vi "LAcontroller.vi"() -> ()   [LabVIEW 2016]
uses:
  controls/FPGAVIreferenceTypeDef.ctl
  controls/Enum.ctl
  controls/FPGAVIreferenceTypeDefScanEngine.ctl
  Course Project/support/Message Queue/Message Cluster.ctl
  controls/EnumFGVHDT.ctl
  <vilib>/rvi/errors/niLvFpgaAdjustHostInterfaceError.vi
  <vilib>/rvi/interface/common/niFpgaWaitOnOcc.vi
  <vilib>/regexp/Match Regular Expression.xnode
  <vilib>/rvi/interface/nirviReadWriteControl/nirviReadWriteControl.xnode
  FPGA Bitfiles/qnmController797_usbRIO_controllerFPGAmu.lvbitx
  <vilib>/rvi/interface/nirviMethod/nirviMethod.xnode
  Course Project/support/Message Queue/Message Queue.lvlib
  <vilib>/rvi/errors/niLvFpgaMergeErrorWithErrorCode.vi
  NiFpgaLv.dll
  <vilib>/FPGAPlugInAG/USB-7856R OEM/niLvFpga_ConfigureFifo_USB-7856R OEM.vi
  <vilib>/FPGAPlugInAG/USB-7856R OEM/niLvFpga_ReadFifo_USB-7856R OEM.vi
panel:
  in  "disable Filters":bool
  out "Warning":string
  in  "setUnityFilters":bool
  out "idSourceName":string
  in  "Identification Type":T1
  out "axialFiltersLoaded":bool
  out "lateralFiltersLoaded":bool
  out "Nominal Response Phi":cluster{dbl[], dbl[]}[](graph)
  out "Nominal Response A":cluster{dbl[], dbl[]}[](graph)
  out "Measured Resp Phi":cluster{dbl[], dbl[]}(graph)
  out "Measured Resp A":cluster{dbl[], dbl[]}(graph)
  out "Time domain":i16[][](graph)
  out "acquisitionDone":dbl(slide) scale=0.0..1.0
  out "Message":string="Exit"
  in  "Filtering mode":enum16{"Axial", "Lateral"}(ring)
  in  "Controller Order":dbl=10.0 min=2.0 max=16.0 step=2.0
  in  "Save identification":bool
  in  "resetFilters":bool
  out "Sampling Frequency":dbl=686813.0 format="%#_4p"
  in  "clearBuffer":bool
  in  "System ID Parameters":T2={"Output Decimation"=1, "Repetitions"=100, "PRBS Order"=12, "low Value"=0.0, "high Value"=0.0005035400390625} {"high Value" format="%#_3p"; "Output Decimation" min=1}
  in  "doControlDesign":bool
  in  "Desired bandwidth":dbl=7000.0 min=500.0 format="%#_13pHz"
  out "Ki":dbl format="%#_3p"
  out "Kp":dbl format="%#_3p"
  out "PRBS length":u16=8191
  # "System Settings"
  # "Control Design"
  # "Measured System Response"
  # "Nominal System Response"
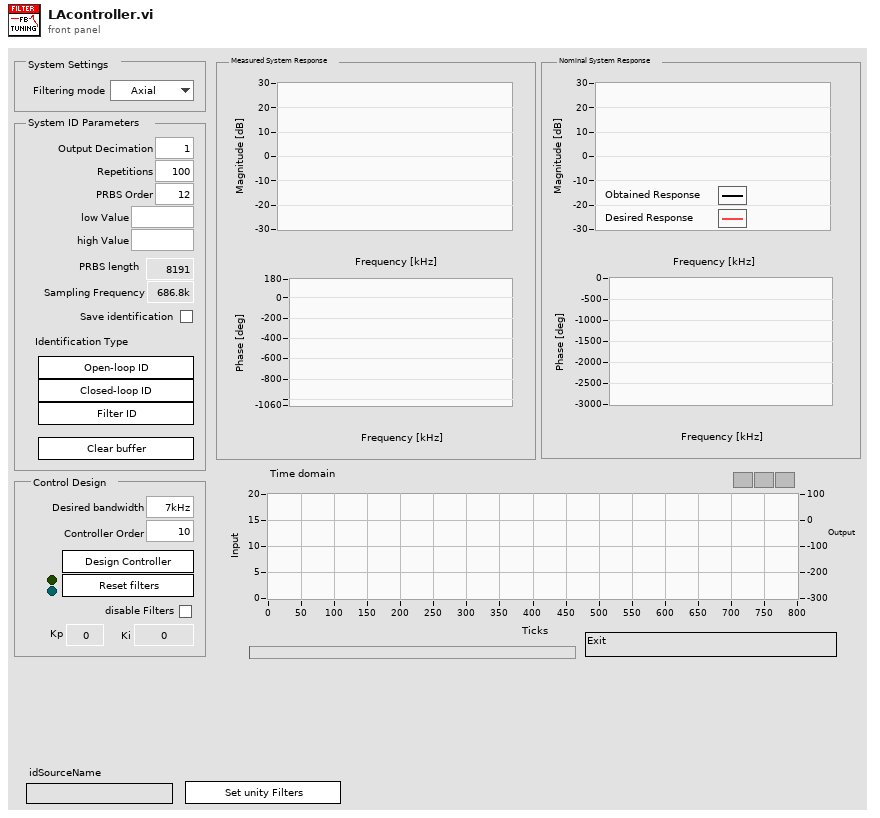
[diagram p1: front panel]
types:
  T1 = cluster{"Error":bool, "Height":bool, "Filter":bool}
  T2 = cluster{"Output Decimation":u16, "Repetitions":u16, "PRBS Order":u16, "low Value":fxp<+/-,17,1>, "high Value":fxp<+/-,17,1>}
  T3 = typedef "Message Queue.lvlib/All Message Queues.ctl" = cluster{"IU":refnum<queue>}
  T4 = cluster{"OldVal":enum16{"Axial", "Lateral"}, "NewVal":enum16{"Axial", "Lateral"}}
  T5 = typedef "eventsource.ctl" = u32
  T6 = cluster{"openLoopID":bool, "closedLoopID":bool, "filterID":bool}
  T7 = typedef "FPGAVIreferenceTypeDefScanEngine.ctl" = refnum<k20>
  T8 = typedef "Enum.ctl" = enum16{"Init", "Read", "Write"}
  T9 = typedef "FPGAVIreferenceTypeDef.ctl" = refnum<k20>
  T10 = cluster{"Output Decimation":u16, "Repetitions":u16, "PRBS Order":u16, "low Value":fxp<+/-,17,1>, "high Value":fxp<+/-,17,1>}[]
  T11 = typedef "Message Queue.lvlib/Message Cluster.ctl" = cluster{"Message":string, "Données de message":variant}
  T12 = cluster{"sysIdOutputRate":u16, "sysIdWaveSize":u16, "sysIdRepetitions":u16, "lowValue":fxp<+/-,16,1>, "highValue":fxp<+/-,16,1>}
  T13 = typedef "EnumFGVHDT.ctl" = enum16{"Init", "Read", "Write", "Push", "Pop"}
  T14 = cluster{"OwnerVi":string, "hdt.int.s.transferSource":u8, "Used":bool}
  T15 = cluster{"scanEngineHz":u32, "feedbackHz":u32, "sicmHz":u32, "rampHz":u32}
  T16 = cluster{"hdt.int.s.transferSource":u8, "hdt.int.p.useInternalMemStartPos":bool, "hdt.int.p.memStartPos":fxp<+,14,14>, "hdt.int.p.readLength":u16, "hdt.int.p.readFwd":bool, "hdt.int.p.memReadDec":u16, "hdt.int.p.startTransfer":bool}
  T17 = cluster{"System ID Parameters":cluster{"Output Decimation":u16, "Repetitions":u16, "PRBS Order":u16, "low Value":fxp<+/-,17,1>, "high Value":fxp<+/-,17,1>}, "PRBS length":u16, "Sampling Frequency":dbl, "flt.p.b8x":fxp<+/-,24,8>[], "flt.p.anot8x":fxp<+/-,24,8>[], "flt.bypass1":bool[]}
  T18 = typedef "imagedata.ctl" = cluster{"image type":i32, "image depth":i32, "image":u8[], "mask":u8[], "colors":u32[], "Rectangle":cluster{"left":i16, "top":i16, "right":i16, "bottom":i16}}
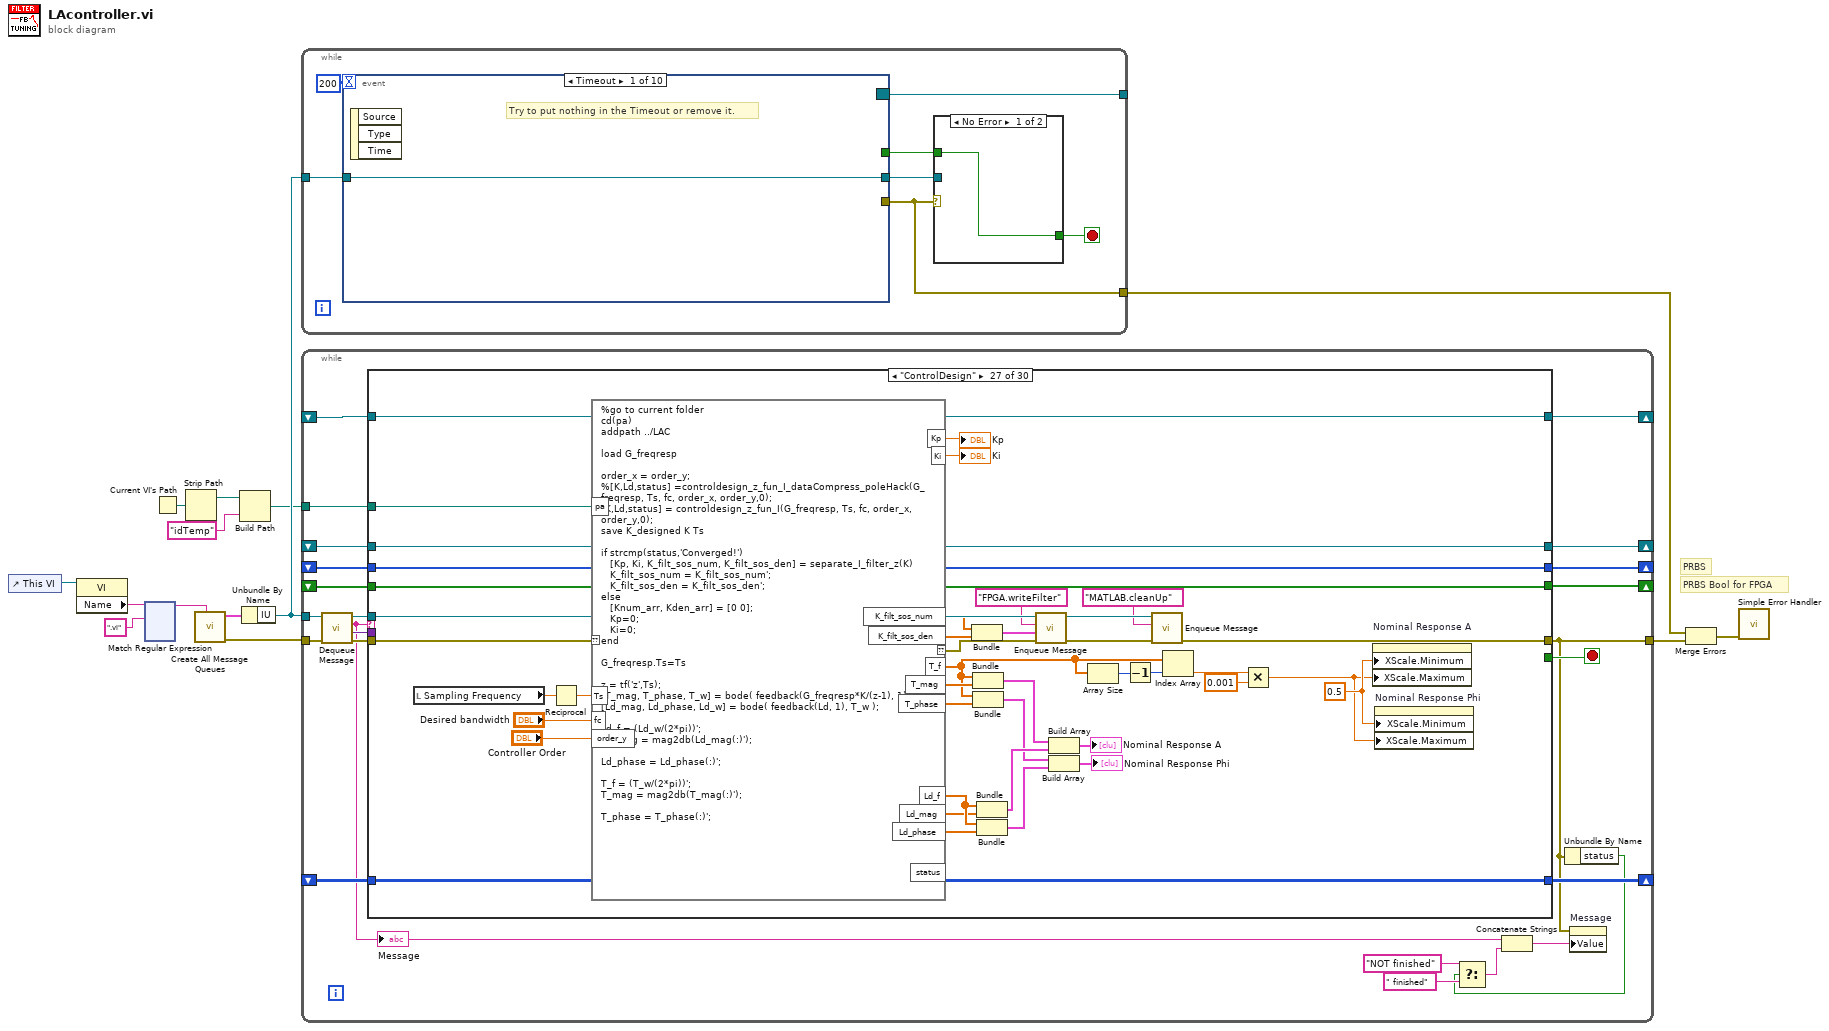
[diagram p0: block diagram]
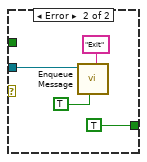
[diagram p2: hidden frame]
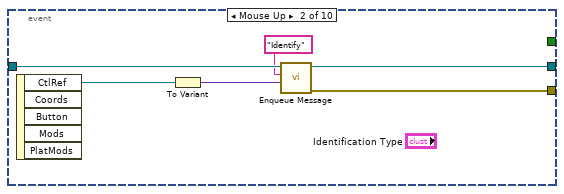
[diagram p3: hidden frame]
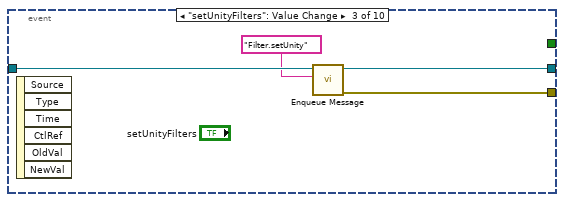
[diagram p4: hidden frame]
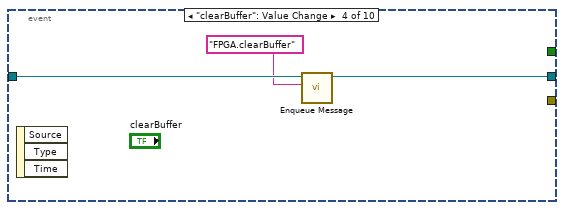
[diagram p5: hidden frame]
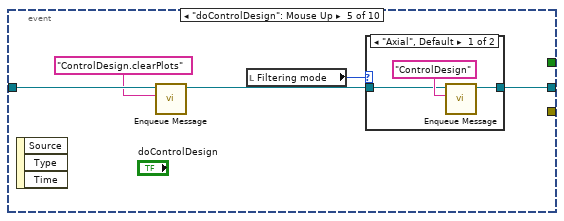
[diagram p6: hidden frame]
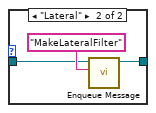
[diagram p7: hidden frame]
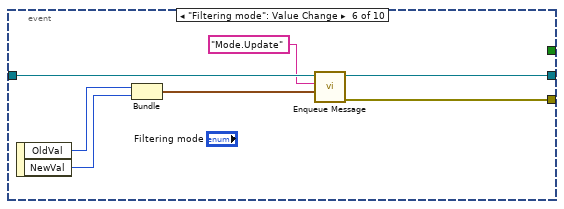
[diagram p8: hidden frame]
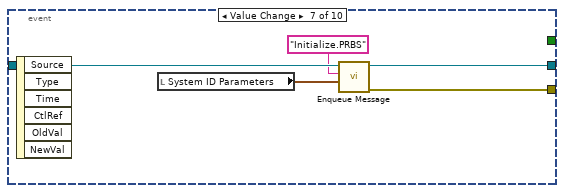
[diagram p9: hidden frame]
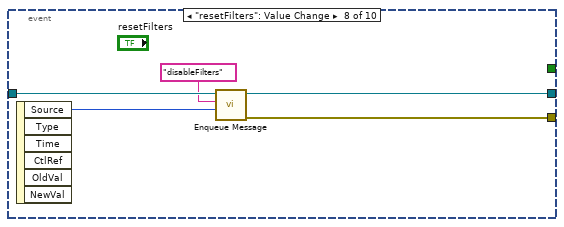
[diagram p10: hidden frame]
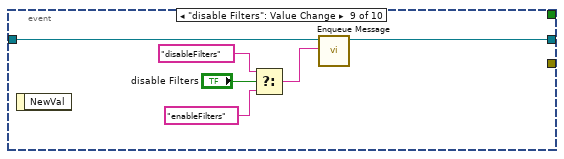
[diagram p11: hidden frame]
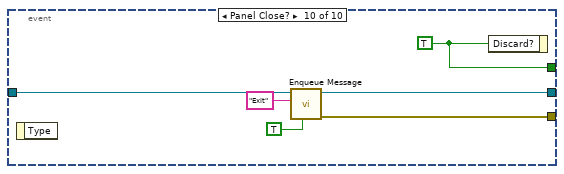
[diagram p12: hidden frame]
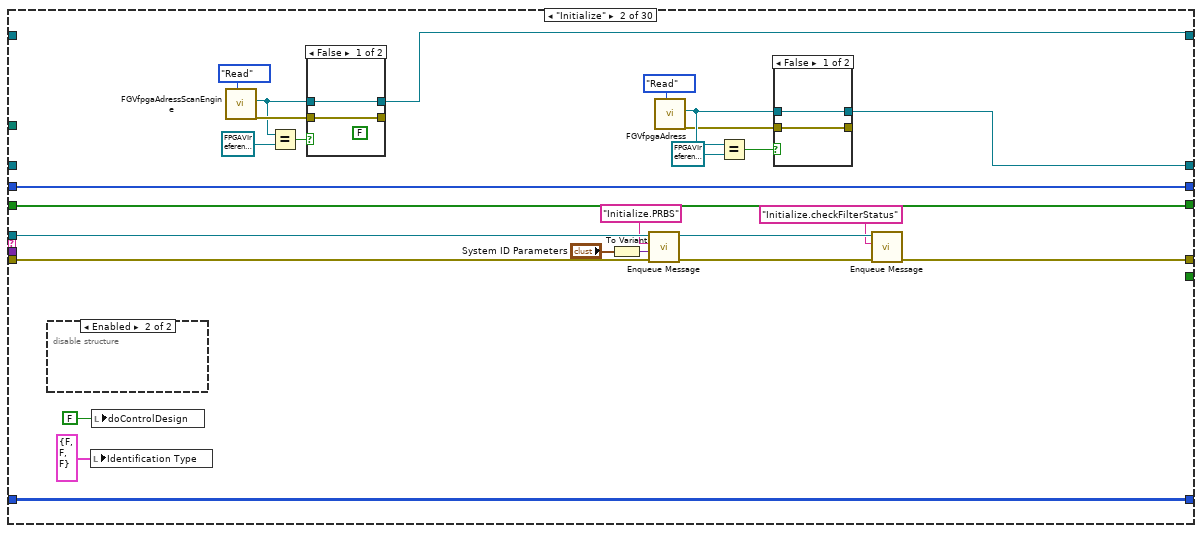
[diagram p14: hidden frame]
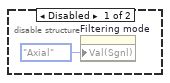
[diagram p15: hidden frame]
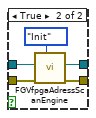
[diagram p16: hidden frame]
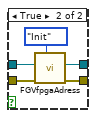
[diagram p17: hidden frame]
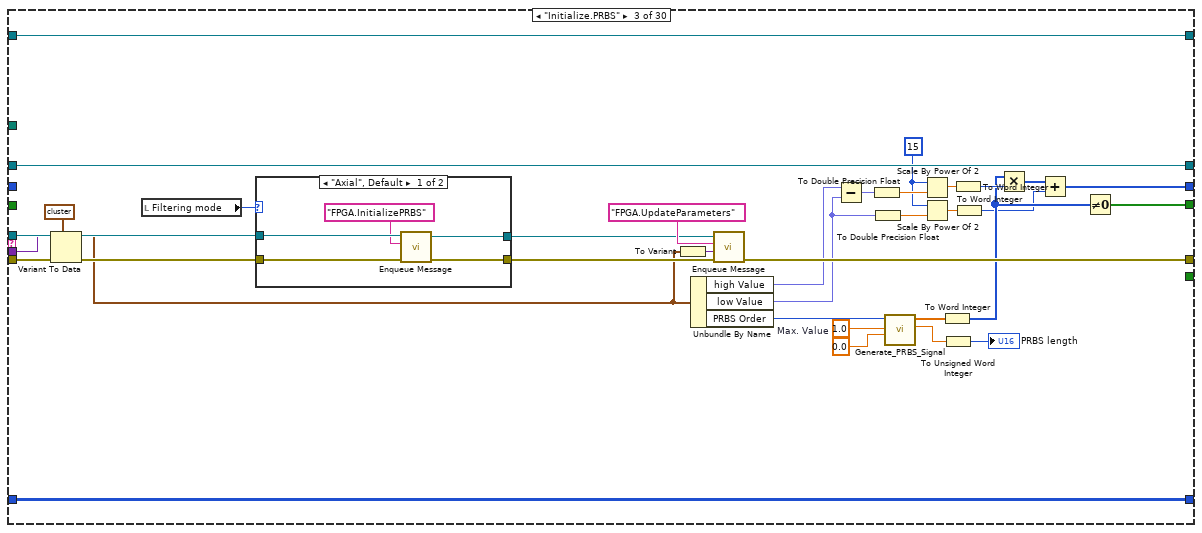
[diagram p18: hidden frame]
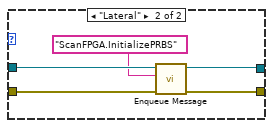
[diagram p19: hidden frame]
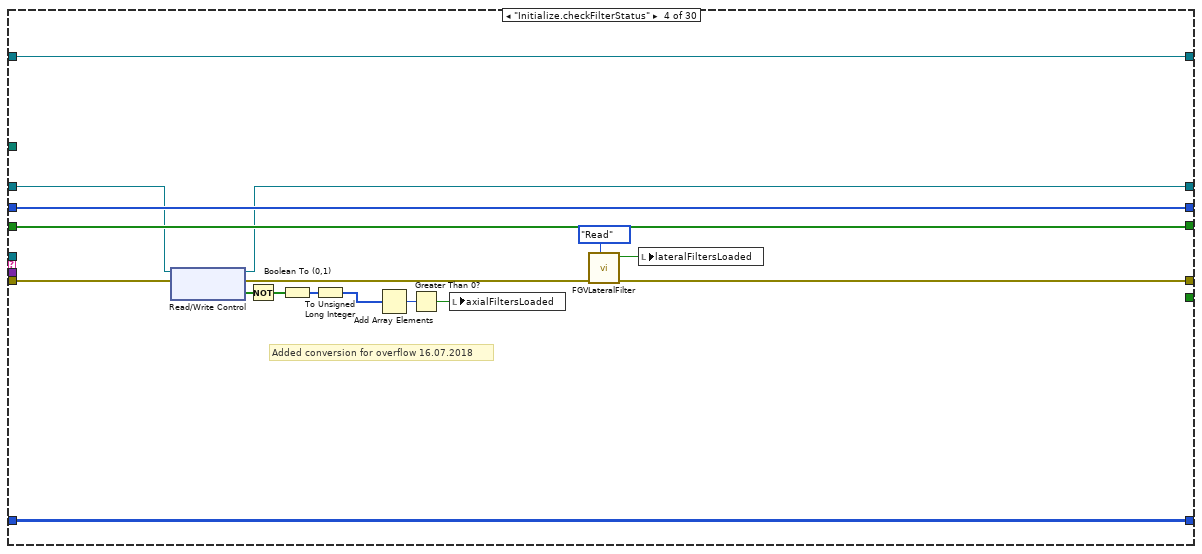
[diagram p20: hidden frame]
diagram:
  # "PRBS Bool for FPGA"
  # "PRBS"
  n1 = control-ref of="This VI"() -> (w4:refnum<vi>)
  n2 = property class="VI"(reference=w4) -> ("Name"=w3:string)  [unwired: 1 in, 2 out]
  n3 = xnode "Match Regular Expression"("input string"=w3, "regular expression"=".vi") -> ("before match"=w1:string)  [unwired: 4 in, 4 out]
  n4 = Current VI's Path() -> (path=w8:path)
  n5 = Strip Path(path=w8) -> (stripped path=w6:path)  [unwired: 1 out]
  n6 = call "Create All Message Queues.vi"("QueueName"=w1) -> ("ErrorOut"=w12:errorcluster, "MessageQueueOut"=w14:T3)  [unwired: 9 in]
  n7 = Build Path(base path=w6, name or relative path="idTemp") -> (appended path=w5:path)
  n8 = Unbundle By Name(w14) -> ("IU"=w13:refnum<queue>)
  n9 = while {
    tunnel: w13 -> [w21]
    tunnel: [w17] -> w9
    tunnel: [w16] -> _
    stop <- w19 stop-if-true
    n10 = event shown="[0] Timeout" {
      selector: _ -> [_ _ _ _ _ _ _ _ _ _]
      dyn-events: [_ _ _ _ _ _ _ _ _ _] -> w16
      timeout: 200 -> [_ _ _ _ _ _ _ _ _ _]
      tunnel: [_ _ _ _ _ _ _ _ _ w80] -> w20
      tunnel: w21 -> [w27 w33 w37 w40 w43 w58 w63 w68 w74 w79]
      tunnel: [_ w28 w35 _ _ w52 w62 w66 _ w78] -> w17
      tunnel: [w27 w29 w36 w39 w45 w53 w60 w64 w73 w77] -> w18
      event Timeout {
        # "Try to put nothing in the Timeout or remove it."
        n11 = event-data() -> ()  [unwired: 1 in, 3 out]
      }
      event "Identification Type.Error", "Identification Type.Height", "Identification Type.Filter": Mouse Up {
        n12 = event-data() -> ("CtlRef"=w31:refnum<vi>)  [unwired: 1 in, 4 out]
        n13 = To Variant(anything=w31) -> (Variant=w30:variant)
        n14 = call "Enqueue Message.vi"("Data"=w30, "Message"="Identify", "Queue"=w33) -> ("error out"=w28:errorcluster, "Queue dup."=w29:refnum<queue>)  [unwired: 7 in]
      }
      event "setUnityFilters": Value Change {
        n15 = event-data() -> ()  [unwired: 1 in, 6 out]
        n16 = call "Enqueue Message.vi"("Message"="Filter.setUnity", "Queue"=w37) -> ("error out"=w35:errorcluster, "Queue dup."=w36:refnum<queue>)  [unwired: 8 in]
      }
      event "clearBuffer": Value Change {
        n17 = event-data() -> ()  [unwired: 1 in, 3 out]
        n18 = call "Enqueue Message.vi"("Message"="FPGA.clearBuffer", "Queue"=w40) -> ("Queue dup."=w39:refnum<queue>)  [unwired: 8 in, 1 out]
      }
      event "doControlDesign": Mouse Up {
        n19 = event-data() -> ()  [unwired: 1 in, 3 out]
        n20 = call "Enqueue Message.vi"("Message"="ControlDesign.clearPlots", "Queue"=w43) -> ("Queue dup."=w42:refnum<queue>)  [unwired: 8 in, 1 out]
        n21 = local read "Filtering mode"() -> (w44:enum16{"Axial", "Lateral"})
        n22 = case shown="\"Axial\", Default" w44 {
          tunnel: w42 -> [w47 w50]
          tunnel: [w46 w49] -> w45
          frame "Axial", Default {
            n23 = call "Enqueue Message.vi"("Message"="ControlDesign", "Queue"=w47) -> ("Queue dup."=w46:refnum<queue>)  [unwired: 8 in, 1 out]
          }
          frame "Lateral" {
            n24 = call "Enqueue Message.vi"("Message"="MakeLateralFilter", "Queue"=w50) -> ("Queue dup."=w49:refnum<queue>)  [unwired: 8 in, 1 out]
          }
        }
      }
      event "Filtering mode": Value Change {
        n25 = event-data() -> ("OldVal"=w55:enum16{"Axial", "Lateral"}, "NewVal"=w56:enum16{"Axial", "Lateral"})  [unwired: 1 in]
        n26 = Bundle("OldVal"=w55, "NewVal"=w56) -> (w54:T4)  [unwired: 1 in]
        n27 = call "Enqueue Message.vi"("Data"=w54, "Message"="Mode.Update", "Queue"=w58) -> ("error out"=w52:errorcluster, "Queue dup."=w53:refnum<queue>)  [unwired: 7 in]
      }
      event "System ID Parameters.PRBS Order": Value Change {
        n28 = event-data() -> ()  [unwired: 1 in, 6 out]
        n29 = local read "System ID Parameters"() -> (w59:T2)
        n30 = call "Enqueue Message.vi"("Data"=w59, "Message"="Initialize.PRBS", "Queue"=w63) -> ("error out"=w62:errorcluster, "Queue dup."=w60:refnum<queue>)  [unwired: 7 in]
      }
      event "resetFilters": Value Change {
        n31 = event-data() -> ("Source"=w67:T5)  [unwired: 1 in, 5 out]
        n32 = call "Enqueue Message.vi"("Data"=w67, "Message"="disableFilters", "Queue"=w68) -> ("error out"=w66:errorcluster, "Queue dup."=w64:refnum<queue>)  [unwired: 7 in]
      }
      event "disable Filters": Value Change {
        n33 = event-data() -> ()  [unwired: 1 in, 1 out]
        n34 = Select(t="disableFilters", s="disable Filters", f="enableFilters") -> (s? t:f=w72:string)
        n35 = call "Enqueue Message.vi"("Message"=w72, "Queue"=w74) -> ("Queue dup."=w73:refnum<queue>)  [unwired: 8 in, 1 out]
      }
      event Panel Close? {
        w80 = TRUE ("Rejeter ?")
        n36 = event-data() -> ()  [unwired: 1 in, 1 out]
        n37 = call "Enqueue Message.vi"("Prioritary message"=TRUE ("Message prioritaire ? (F)"), "Message"="Exit", "Queue"=w79) -> ("error out"=w78:errorcluster, "Queue dup."=w77:refnum<queue>)  [unwired: 7 in]
        n38 = event-data ("Event Filter Node")("Discard?"=w80) -> ()  [unwired: 1 in, 1 out]
      }
    }
    n39 = case shown="No Error" w17 {
      tunnel: [w22 TRUE ("Rejeter ?")] -> w19
      tunnel: w20 -> [w22 _]
      tunnel: w18 -> [_ w25]
      frame No Error {
      }
      frame Error {
        n40 = call "Enqueue Message.vi"("Prioritary message"=TRUE ("Message prioritaire ? (F)"), "Message"="Exit", "Queue"=w25) -> ()  [unwired: 7 in, 2 out]
      }
    }
  }
  n41 = while {
    tunnel: w13 -> [w99]
    tunnel: w12 -> [w103]
    tunnel: [w85] -> w10
    shift-right: [w97] -> _
    shift-left: _ -> [w98]
    shift-right: [w96] -> _
    shift-left: _ -> [w95]
    shift-right: [w94] -> _
    shift-left: _ -> [w93]
    shift-right: [w91] -> _
    shift-left: _ -> [w92]
    shift-right: [w90] -> _
    shift-left: _ -> [w89]
    tunnel: w5 -> [w88]
    stop <- w104 stop-if-true
    n42 = call "Dequeue Message.vi"("entrée d'erreur (pas d'erreur)"=w103, "File d'attente de messages"=w99) -> ("sortie d'erreur"=w102:errorcluster, "Données de message"=w101:variant, "Message"=w87:string, "File d'attente de message dup."=w100:refnum<queue>)  [unwired: 6 in]
    "Message" <- w87
    n43 = case "Conditions des messages" shown="\"ControlDesign\"" w87 {
      selector: w87 -> [_ _ _ _ _ _ _ _ _ _ _ _ _ _ _ _ _ _ _ _ _ _ _ _ _ _ _ _ _ w1015]
      tunnel: w100 -> [_ w133 w184 _ _ w235 w254 w341 w365 _ _ _ _ _ _ _ _ _ _ _ _ _ w793 _ _ _ w970 _ w1006 _]
      tunnel: w102 -> [w110 w132 w181 w209 w219 w234 w261 w336 w353 w373 w385 w404 w428 w451 w520 w550 w592 w630 w689 w718 w728 w752 w760 w831 w879 w927 w935 w995 w1004 _]
      tunnel: [w110 w114 w185 w200 w219 w223 w280 w323 w352 w373 w375 w400 w438 w459 w527 w547 w591 w631 w654 w702 w731 w752 w761 w830 w868 w927 w931 w995 w1003 w1013] -> w85
      tunnel: [_ _ _ _ _ _ _ _ _ _ _ _ _ _ _ _ _ _ _ _ _ _ _ _ _ _ _ _ TRUE _] -> w104
      tunnel: w101 -> [_ _ w180 _ _ w229 _ w335 _ _ _ w403 _ _ w519 w549 _ _ w690 _ _ _ w775 _ w878 _ _ _ _ _]
      tunnel: w98 -> [w109 _ w171 w208 w218 w233 w283 w322 w364 w372 w381 w402 w437 w465 w516 w545 w594 w628 w679 w717 w733 w751 w812 w836 w852 w926 w969 w994 w1002 w1011]
      tunnel: [w109 w117 w171 w207 w218 w233 w283 w321 w364 w372 w374 w401 w436 w460 w526 w544 w593 w629 w675 w704 w732 w751 w812 w836 w852 w926 w969 w994 w1002 w1011] -> w97
      tunnel: [w108 w136 w168 w213 w217 w232 w287 w340 w363 w371 w377 w415 w430 w464 w525 w553 w590 w627 w693 w722 w735 w750 w811 w835 w885 w925 w968 w993 w1001 w1010] -> w96
      tunnel: w95 -> [w108 w136 _ w213 w217 w232 w287 w340 w363 w371 w377 w415 w430 w464 w525 w553 w590 w627 w693 w722 w735 w750 w811 w835 w885 w925 w968 w993 w1001 w1010]
      tunnel: [w107 w135 w182 w212 w216 w222 w279 w339 w362 w370 w384 w414 w433 w463 w524 w552 w588 w625 w692 w721 w734 w749 w810 w834 w884 w924 w967 w992 w1000 w1009] -> w94
      tunnel: w93 -> [w107 w135 w182 w212 w216 w222 w279 w339 w362 w370 w384 w414 w433 w463 w524 w552 _ _ w692 w721 w734 w749 w810 w834 w884 w924 w967 w992 w1000 w1009]
      tunnel: w92 -> [w106 _ w177 w211 w215 w231 w278 w338 w361 w369 w380 w398 w440 w462 w522 w543 w587 w637 w681 w720 w730 w748 w813 w833 w883 w923 w942 w990 w998 w1008]
      tunnel: [w106 w118 w177 w211 w215 w231 w278 w338 w361 w369 w380 w397 w439 w462 w521 w543 w587 w637 w681 w720 w730 w748 w813 w833 w883 w923 w942 w990 w998 w1008] -> w91
      tunnel: [w105 w134 w170 w210 w214 w230 w286 w337 w360 w368 w378 w413 w431 w461 w523 w551 w595 w636 w680 w719 w729 w747 w797 w832 w882 w922 w941 w989 w999 w1007] -> w90
      tunnel: w89 -> [w105 w134 _ w210 w214 w230 w286 w337 w360 w368 w378 w413 w431 w461 w523 w551 w595 w636 w680 w719 w729 w747 w797 w832 w882 w922 w941 w989 w999 w1007]
      tunnel: w88 -> [_ _ _ _ _ _ _ _ _ _ _ _ _ _ _ _ _ _ _ _ _ _ w791 _ w860 _ w937 w972 _ _]
      frame "--------- Initialization ---------" {
      }
      frame "Initialize" {
        n44 = disable-structure shown="Enabled" {
          frame Disabled {
            n45 = property on="Filtering mode" class="Enum (strict)"("Val(Sgnl)"=enum16{"Axial", "Lateral"}."Axial" ("Filtering mode")) -> ()  [unwired: 2 in, 2 out]
          }
          frame Enabled {
          }
        }
        n46 = local write "Identification Type"(T6 {"openLoopID"=FALSE, "closedLoopID"=FALSE, "filterID"=FALSE} ("Identification Type")) -> ()
        n47 = local write "doControlDesign"(FALSE ("doLatFilterDesign")) -> ()
        n48 = call "FGVfpgaAdressScanEngine.vi"("Enum"=Enum."Read") -> ("error out"=w127:errorcluster, "FPGA.SEout"=w125:T7)  [unwired: 6 in, 3 out]
        n49 = Equal?(x=w125, y=T7 refnum ("FPGA.SEout")) -> (x = y?=w126:bool)
        n50 = case shown="False" w126 {
          tunnel: [w139 w144] -> w118
          tunnel: [w138 w143] -> _
          tunnel: w127 -> [w138 w142]
          tunnel: w125 -> [w139 w141]
          frame False {
            (unwired) FALSE
          }
          frame True {
            n51 = call "FGVfpgaAdressScanEngine.vi"("Enum"=Enum."Init", "error in"=w142, "FPGA.SEin"=w141) -> ("error out"=w143:errorcluster, "FPGA.SEout"=w144:T7)  [unwired: 4 in, 3 out]
          }
        }
        n52 = To Variant(anything="System ID Parameters") -> (Variant=w111:variant)
        n53 = call "Enqueue Message.vi"("error in"=w132, "Data"=w111, "Message"="Initialize.PRBS", "Queue"=w133) -> ("error out"=w115:errorcluster, "Queue dup."=w116:refnum<queue>)  [unwired: 6 in]
        n54 = call "FGVfpgaAdress.vi"("Enum"=Enum."Read") -> ("error out"=w119:errorcluster, "FPGA VI Reference Out"=w121:T9)  [unwired: 5 in, 4 out]
        n55 = Equal?(x=w121, y=T9 refnum ("FPGA VI Reference Out")) -> (x = y?=w120:bool)
        n56 = case shown="False" w120 {
          tunnel: [w146 w151] -> w117
          tunnel: [w145 w150] -> _
          tunnel: w119 -> [w145 w149]
          tunnel: w121 -> [w146 w148]
          frame False {
          }
          frame True {
            n57 = call "FGVfpgaAdress.vi"("Enum"=Enum."Init", "error in"=w149, "FPGA VI Reference In"=w148) -> ("error out"=w150:errorcluster, "FPGA VI Reference Out"=w151:T9)  [unwired: 3 in, 4 out]
          }
        }
        n58 = call "Enqueue Message.vi"("error in"=w115, "Message"="Initialize.checkFilterStatus", "Queue"=w116) -> ("error out"=w114:errorcluster)  [unwired: 7 in, 1 out]
      }
      frame "Initialize.PRBS" {
        w159 = i16 15 ("n")
        w178 = 1.0  # Max. Value
        n59 = Variant To Data(error in=w181, type=T2 {"Output Decimation"=1, "Repetitions"=1000, "PRBS Order"=12, "low Value"=0.0, "high Value"=0.0005035400390625} ("System ID Parameters"), Variant=w180) -> (data=w154:T2, error out=w164:errorcluster)
        n60 = local read "Filtering mode"() -> (w153:enum16{"Axial", "Lateral"})
        n61 = case shown="\"Axial\", Default" w153 {
          tunnel: [w191 w193] -> w186
          tunnel: w184 -> [w190 w196]
          tunnel: [w189 w194] -> w152
          tunnel: w164 -> [w187 w192]
          frame "Axial", Default {
            n62 = call "Enqueue Message.vi"("error in"=w187, "Message"="FPGA.InitializePRBS", "Queue"=w190) -> ("error out"=w191:errorcluster, "Queue dup."=w189:refnum<queue>)  [unwired: 7 in]
          }
          frame "Lateral" {
            n63 = call "Enqueue Message.vi"("error in"=w192, "Message"="ScanFPGA.InitializePRBS", "Queue"=w196) -> ("error out"=w193:errorcluster, "Queue dup."=w194:refnum<queue>)  [unwired: 7 in]
          }
        }
        n64 = To Variant(anything=w154) -> (Variant=w155:variant)
        n65 = Unbundle By Name(w154) -> ("high Value"=w173:fxp<+/-,17,1>, "low Value"=w161:fxp<+/-,17,1>, "PRBS Order"=w160:u16)
        n66 = call "Enqueue Message.vi"("error in"=w186, "Data"=w155, "Message"="FPGA.UpdateParameters", "Queue"=w152) -> ("error out"=w185:errorcluster)  [unwired: 6 in, 1 out]
        n67 = Subtract(x=w173, y=w161) -> (x-y=w176:fxp<+/-,18,2>)
        n68 = To Double Precision Float(number=w176) -> (double precision float=w162:dbl)
        n69 = To Double Precision Float(number=w161) -> (double precision float=w163:dbl)
        n70 = call "Generate_PRBS_Signal.vi"("Min.Value"=0.0, "Max. Value"=w178, "PRBS Order"=w160) -> ("PRBS Signal Length"=w169:dbl, "PRBS Signal"=w183:dbl[])  [unwired: 7 in]
        n71 = Scale By Power Of 2(n=w159, x=w162) -> (x*2^n=w175:dbl)
        n72 = Scale By Power Of 2(n=w159, x=w163) -> (x*2^n=w167:dbl)
        n73 = To Word Integer(number=w183) -> (16bit integer=w172:i16[])
        n74 = To Unsigned Word Integer(number=w169) -> (unsigned 16bit integer=→"PRBS length":u16)
        n75 = To Word Integer(number=w175) -> (16bit integer=w174:i16)
        n76 = To Word Integer(number=w167) -> (16bit integer=w166:i16)
        n77 = Multiply(x=w172, y=w174) -> (x*y=w165:i16[])
        n78 = Add(x=w165, y=w166) -> (x+y=w168:i16[])
        n79 = Not Equal To 0?(x=w172) -> (x != 0?=w170:bool[])
      }
      frame "Initialize.checkFilterStatus" {
        # "Added conversion for overflow 16.07.2018"
        n80 = xnode "Read/Write Control"("FPGA VI Reference In"=w208, "error in"=w209) -> ("FPGA VI Reference Out"=w207:T9, "error out"=w201:errorcluster, "flt.bypass1"=w206:bool[])
        n81 = Not(x=w206) -> (.not. x?=w204:bool[])
        n82 = Boolean To (0,1)(Boolean=w204) -> (0, 1=w205:i16[])
        n83 = To Unsigned Long Integer(number=w205) -> (unsigned 32bit integer=w197:u32[])
        n84 = Add Array Elements(numeric array=w197) -> (sum=w203:u32)
        n85 = Greater Than 0?(x=w203) -> (x > 0?=w202:bool)
        n86 = local write "axialFiltersLoaded"(w202) -> ()
        n87 = call "FGVLateralFilter.vi"("Enum"=Enum."Read", "error in"=w201) -> ("error out"=w200:errorcluster, "Filter valid output"=w198:bool)  [unwired: 5 in, 1 out]
        n88 = local write "lateralFiltersLoaded"(w198) -> ()
      }
      frame "--- Modal ----" {
      }
      frame "Mode.Update" {
        n89 = Variant To Data(type=T4 {"OldVal"=enum."Axial", "NewVal"=enum."Axial"} ("output cluster"), Variant=w229) -> (data=w227:T4)  [unwired: 1 in, 1 out]
        n90 = local read "System ID Parameters"() -> (w221:T2)
        n91 = local read "Desired bandwidth"() -> (w220:dbl)
        n92 = Unbundle(w227) -> ("OldVal"=w225:enum16{"Axial", "Lateral"}, "NewVal"=w224:enum16{"Axial", "Lateral"})
        n93 = Not Equal?(x=w225, y=w224) -> (x != y?=w226:bool)
        n94 = case shown="True" w226 {
          tunnel: w225 -> [_ w239]
          tunnel: w224 -> [_ w252]
          tunnel: w234 -> [w236 w249]
          tunnel: [w236 w248] -> w223
          tunnel: w235 -> [_ w251]
          tunnel: w221 -> [_ w238]
          tunnel: w220 -> [_ w237]
          frame False {
          }
          frame True {
            # "Initial desired frequencies"
            # "Initial sysID params"
            n95 = feedback #1(T10 [{"Output Decimation"=1, "Repetitions"=100, "PRBS Order"=12, "low Value"=0.0, "high Value"=0.00140380859375}, {"Output Decimation"=80, "Repetitions"=100, "PRBS Order"=12, "low Value"=0.0, "high Value"=0.0005035400390625}]) -> (w244:T10)
            n96 = Replace Array Subset(array=w244, new element=w238, index=w239) -> (w245:T10)
            n97 = feedback-in #1(w245) -> ()
            n98 = Index Array(array=w244, index=w252) -> (element=w247:T2)
            n99 = local write "System ID Parameters"(w247) -> ()
            n100 = call "Enqueue Message.vi"("error in"=w249, "Data"=w247, "Message"="Initialize.PRBS", "Queue"=w251) -> ("error out"=w248:errorcluster)  [unwired: 6 in, 1 out]
            n101 = feedback #2(dbl[] [8000.0, 1000.0]) -> (w243:dbl[])
            n102 = Replace Array Subset(array=w243, new element=w237, index=w239) -> (w242:dbl[])
            n103 = Index Array(array=w243, index=w252) -> (element=w241:dbl)
            n104 = feedback-in #2(w242) -> ()
            n105 = local write "Desired bandwidth"(w241) -> ()
          }
        }
      }
      frame "doIdentification" {
        # "Z controller VI ready\n(engaged)"
        n106 = while {
          tunnel: w261 -> [w309]
          tunnel: [w308] -> w253
          stop <- w306 stop-if-true
          n107 = call "FGVTriggerQueue.vi"("Enum"=Enum."Read", "error in"=w309) -> ("error out"=w308:errorcluster, "Ready OUT?"=w306:bool)  [unwired: 8 in]
          n108 = Wait (ms)(milliseconds to wait=u32 10) -> ()  [unwired: 1 out]
        }
        n109 = disable-structure shown="FPGA_BUILT==PXI_7975R, Default" {
          disable-tunnel: [w302 w304] -> w258
          disable-tunnel: w254 -> [w301 w304]
          disable-tunnel: w253 -> [w300 w303]
          disable-tunnel: [w299 w303] -> w256
          frame condition #0 (active) {
            n110 = call "Enqueue Message.vi"("error in"=w300, "Data"=TRUE, "Message"="Buffer", "Queue"=w301) -> ("error out"=w299:errorcluster, "Queue dup."=w302:refnum<queue>)  [unwired: 6 in]
          }
          frame condition #1 {
          }
        }
        n111 = local read "Filtering mode"() -> (w259:enum16{"Axial", "Lateral"})
        n112 = local read "System ID Parameters"() -> (w277:T2)
        n113 = call "Enqueue Message.vi"("error in"=w256, "Message"="FPGA.clearBuffer", "Queue"=w258) -> ("error out"=w288:errorcluster, "Queue dup."=w257:refnum<queue>)  [unwired: 7 in]
        n114 = Equal?(x=w259, y=enum16{"Axial", "Lateral"}."Axial" ("x")) -> (x = y?=w263:bool)
        n115 = call "Enqueue Message.vi"("error in"=w288, "Data"=w259, "Message"="FPGA.startId", "Queue"=w257) -> ("error out"=w271:errorcluster, "Queue dup."=w282:refnum<queue>)  [unwired: 6 in]
        n116 = call "FGVSamplingRates.vi"("Enum"=Enum."Read", "error in"=w271) -> ("error out"=w284:errorcluster, "samplingRatesOut"=w266:T15)  [unwired: 8 in]
        n117 = Unbundle By Name(w266) -> ("feedbackHz"=w265:u32)
        n118 = Unbundle By Name(w266) -> ("scanEngineHz"=w267:u32)
        n119 = Unbundle By Name(w277) -> ("Output Decimation"=w275:u16)
        n120 = call "Enqueue Message.vi"("error in"=w284, "Message"="FPGA.readSystemResponse", "Queue"=w282) -> ("error out"=w270:errorcluster, "Queue dup."=w268:refnum<queue>)  [unwired: 7 in]
        n121 = Select(t=w265, s=w263, f=w267) -> (s? t:f=w264:u32)
        n122 = Divide(x=w264, y=w275) -> (x/y=→"Sampling Frequency":dbl)
        n123 = disable-structure shown="FPGA_BUILT==PXI_7975R, Default" {
          disable-tunnel: [w294 w296] -> w285
          disable-tunnel: w270 -> [w293 w295]
          disable-tunnel: [w292 w295] -> w269
          disable-tunnel: w268 -> [w291 w296]
          frame condition #0 (active) {
            n124 = call "Enqueue Message.vi"("error in"=w293, "Data"=FALSE, "Message"="Buffer", "Queue"=w291) -> ("error out"=w292:errorcluster, "Queue dup."=w294:refnum<queue>)  [unwired: 6 in]
          }
          frame condition #1 {
          }
        }
        n125 = control-ref of="Filtering mode"() -> (w262:refnum<vi>)
        n126 = call "Enqueue Message.vi"("error in"=w269, "Data"=w262, "Message"="MATLAB.identFreqResp", "Queue"=w285) -> ("error out"=w280:errorcluster)  [unwired: 6 in, 1 out]
      }
      frame "Identify" {
        # "In ZController, the following sequence is performed:\n- Engage with current gains\n- Set gains Gi=10u Gp = 0\n- Send ready to"
        # "Available ID sources\n0: Error, open-loop\n1: Height, closed-loop\n2: Filter output"
        n127 = Variant To Data(error in=w336, type=refnum<vi> refnum ("CtlRef"), Variant=w335) -> (data=w333:refnum<vi>, error out=w331:errorcluster)
        n128 = property class="Bool (strict)"(reference=w333) -> ("Owner"=w330:refnum<vi>, "Label.Text"=w326:string)  [unwired: 1 in, 2 out]
        n129 = To More Specific Class(target class=refnum<vi> refnum ("Identification Type"), reference=w330, error in=w331) -> (specific class reference=w329:refnum<vi>, error out=w328:errorcluster)
        n130 = property class="Clust (strict)"(reference=w329, error in=w328) -> (error out=w325:errorcluster, "Controls[]"=w327:refnum<vi>[])  [unwired: 1 out]
        n131 = for {
          tunnel: w327 -> [w347] mode=indexing
          tunnel: w326 -> [w346]
          tunnel: [w344] -> w319
          tunnel: [w343] -> w310
          tunnel: [w342] -> w320
          tunnel: w325 -> [w348]
          i -> [w344]
          stop <- w345 stop-if-true
          n132 = property class="Ctl"(reference=w347, error in=w348) -> (error out=w342:errorcluster, "Label.Text"=w343:string)  [unwired: 1 out]
          n133 = Equal?(x=w343, y=w346) -> (x = y?=w345:bool)
        }
        "idSourceName" <- w310
        n134 = xnode "Read/Write Control"("FPGA VI Reference In"=w322, "error in"=w320, "sid.p.idSource"=w319) -> ("FPGA VI Reference Out"=w321:T9, "error out"=w314:errorcluster)
        n135 = Bundle By Name(cluster=T11 {"Message"="ZController.Engage", "Données de message"=variant} ("Cluster Message"), "Données de message"=w310) -> (w311:T11)
        n136 = Obtain Queue(name (unnamed)="ZController", element data type=T11 {"Message"="", "Données de message"=variant} ("Cluster Message"), error in (no error)=w314) -> (queue out=w317:refnum<queue>, error out=w316:errorcluster)  [unwired: 2 in, 1 out]
        n137 = Enqueue Element(queue=w317, element=w311, error in (no error)=w316) -> (error out=w313:errorcluster)  [unwired: 1 in, 2 out]
        n138 = call "Enqueue Message.vi"("error in"=w313, "Message"="doIdentification", "Queue"=w341) -> ("error out"=w323:errorcluster)  [unwired: 7 in, 1 out]
      }
      frame "Filter.setUnity" {
        n139 = local read "Controller Order"() -> (w359:dbl)
        n140 = Divide(x=w359, y=2.0) -> (x/y=w357:dbl)
        n141 = To Long Integer(number=w357) -> (32bit integer=w349:i32)
        n142 = for {
          N: w349 -> [_]
          tunnel: [dbl[] [1.0, 0.0, 0.0]] -> w356 mode=concatenating
          tunnel: [dbl[] [0.0, 0.0]] -> w355 mode=concatenating
          workers-P: _ -> [_]
        }
        n143 = Bundle(w356, w355) -> (w351:cluster{dbl[], dbl[]})  [unwired: 1 in]
        n144 = local write "setUnityFilters"(FALSE ("setUnityFilters")) -> ()
        n145 = call "Enqueue Message.vi"("error in"=w353, "Data"=w351, "Message"="FPGA.writeFilter", "Queue"=w365) -> ("error out"=w352:errorcluster)  [unwired: 6 in, 1 out]
      }
      frame "--- FPGA ---" {
      }
      frame "FPGA.InitializePRBS" {
        n146 = for {
          tunnel: w381 -> [w393]
          tunnel: [w391] -> w383
          tunnel: w385 -> [w390]
          tunnel: [w389] -> w382
          tunnel: w378 -> [w387] mode=indexing
          tunnel: cluster{"write":bool, "data":bool, "index":u16} {"write"=TRUE, "data"=FALSE, "index"=0} ("sid.m.motion") -> [w386]
          i -> [w392]
          n147 = Bundle By Name(cluster=w386, "data"=w387, "index"=w392) -> (w388:cluster{"write":bool, "data":bool, "index":u16})
          n148 = xnode "Read/Write Control"("FPGA VI Reference In"=w393, "error in"=w390, "sid.m.motion"=w388) -> ("FPGA VI Reference Out"=w391:T9, "error out"=w389:errorcluster)
        }
        n149 = xnode "Read/Write Control"("FPGA VI Reference In"=w383, "error in"=w382, "sid.m.motion"=cluster{"write":bool, "data":bool, "index":u16} {"write"=FALSE, "data"=FALSE, "index"=0}) -> ("FPGA VI Reference Out"=w374:T9, "error out"=w375:errorcluster)
      }
      frame "FPGA.UpdateParameters" {
        # "Get a big enough buffer"
        n150 = Variant To Data(error in=w404, type=T2 {"Output Decimation"=1, "Repetitions"=1000, "PRBS Order"=12, "low Value"=0.0, "high Value"=0.0005035400390625} ("System ID Parameters"), Variant=w403) -> (data=w411:T2, error out=w416:errorcluster)
        n151 = Unbundle By Name(w411) -> ("Output Decimation"=w409:u16, "low Value"=w407:fxp<+/-,17,1>, "high Value"=w408:fxp<+/-,17,1>, "Repetitions"=w406:u16)
        n152 = local read "PRBS length"() -> (w405:u16)
        n153 = Bundle By Name(cluster=T12 {"sysIdOutputRate"=0, "sysIdWaveSize"=0, "sysIdRepetitions"=0, "lowValue"=0.0, "highValue"=0.0} ("sid.p.params"), "sysIdWaveSize"=w405, "sysIdOutputRate"=w409, "lowValue"=w407, "highValue"=w408, "sysIdRepetitions"=w406) -> (w394:T12)
        n154 = Multiply(x=w405, y=w406) -> (x*y=w399:u16)
        n155 = xnode "Read/Write Control"("FPGA VI Reference In"=w402, "error in"=w416, "sid.p.params"=w394) -> ("FPGA VI Reference Out"=w417:T9, "error out"=w396:errorcluster)
        n156 = xnode "Read/Write Control"("FPGA VI Reference In"=w398, "error in"=w396, "se.sid.p.params"=w394) -> ("FPGA VI Reference Out"=w397:T7, "error out"=w395:errorcluster)
        n157 = disable-structure shown="FPGA_BUILT==PXI_7975R, Default" {
          disable-tunnel: w417 -> [w422 w427]
          disable-tunnel: w395 -> [w421 w426]
          disable-tunnel: [w420 w425] -> w401
          disable-tunnel: [w419 w424] -> w400
          disable-tunnel: w399 -> [w418 w423]
          frame condition #0 {
            n158 = xnode "Invoke Method"("FPGA VI Reference In"=w422, "error in"=w421, "Requested Depth"=w418) -> ("FPGA VI Reference Out"=w420:T9, "error out"=w419:errorcluster)  [unwired: 1 out]
          }
          frame condition #1 (active) {
            n159 = xnode "Invoke Method"("FPGA VI Reference In"=w427, "error in"=w426, "Requested Depth"=w423) -> ("FPGA VI Reference Out"=w425:T9, "error out"=w424:errorcluster)  [unwired: 1 out]
          }
        }
      }
      frame "ScanFPGA.InitializePRBS" {
        n160 = xnode "Read/Write Control"("FPGA VI Reference In"=w437, "error in"=w428, "sid.allowExternalRecord"=TRUE) -> ("FPGA VI Reference Out"=w436:T9, "error out"=w435:errorcluster)
        n161 = for {
          tunnel: w440 -> [w450]
          tunnel: [w448] -> w442
          tunnel: w435 -> [w447]
          tunnel: [w446] -> w441
          tunnel: w431 -> [w444] mode=indexing
          tunnel: cluster{"write":bool, "index":u16, "data":bool} {"write"=TRUE, "index"=0, "data"=FALSE} ("se.sid.prbs") -> [w443]
          i -> [w449]
          n162 = Bundle By Name(cluster=w443, "data"=w444, "index"=w449) -> (w445:cluster{"write":bool, "index":u16, "data":bool})
          n163 = xnode "Read/Write Control"("FPGA VI Reference In"=w450, "error in"=w447, "se.sid.prbs"=w445) -> ("FPGA VI Reference Out"=w448:T7, "error out"=w446:errorcluster)
        }
        n164 = xnode "Read/Write Control"("FPGA VI Reference In"=w442, "error in"=w441, "se.sid.prbs"=cluster{"write":bool, "index":u16, "data":bool} {"write"=FALSE, "index"=0, "data"=FALSE}) -> ("FPGA VI Reference Out"=w439:T7, "error out"=w438:errorcluster)
      }
      frame "FPGA.clearBuffer" {
        w453 = 10 ("Timeout (ms)")
        w454 = u32 50 ("milliseconds to wait")
        w455 = u32 0 ("Elements Remaining")
        w452 = 5
        n165 = for {
          N: w452 -> [_]
          shift-right: [w488] -> _
          shift-left: w455 -> [w489]
          tunnel: w465 -> [w495]
          tunnel: w451 -> [w494]
          tunnel: [w493] -> w456
          tunnel: [w492] -> w457
          tunnel: w454 -> [w491]
          tunnel: w453 -> [w490]
          n166 = disable-structure shown="FPGA_BUILT==RIO0" {
            disable-tunnel: w495 -> [w502 w509]
            disable-tunnel: w494 -> [w501 w508]
            disable-tunnel: [w500 w507] -> w493
            disable-tunnel: [w499 w506] -> w492
            disable-tunnel: w490 -> [w498 w505]
            disable-tunnel: w489 -> [w497 w504]
            disable-tunnel: [w496 w503] -> w488
            frame condition #0 {
              n167 = xnode "Invoke Method"("FPGA VI Reference In"=w502, "error in"=w501, "Number of Elements"=w497, "Timeout (ms)"=w498) -> ("FPGA VI Reference Out"=w499:T9, "error out"=w500:errorcluster, "Elements Remaining"=w496)  [unwired: 1 out]
            }
            frame condition #1 (active) {
              n168 = xnode "Invoke Method"("FPGA VI Reference In"=w509, "error in"=w508, "Number of Elements"=w504, "Timeout (ms)"=w505) -> ("FPGA VI Reference Out"=w506:T9, "error out"=w507:errorcluster, "Elements Remaining"=w503:u32)  [unwired: 1 out]
            }
          }
          n169 = Wait (ms)(milliseconds to wait=w491) -> ()  [unwired: 1 out]
        }
        n170 = local write "clearBuffer"(FALSE ("clearBuffer")) -> ()
        n171 = for {
          N: w452 -> [_]
          shift-right: [w466] -> _
          shift-left: w455 -> [w467]
          tunnel: w454 -> [w469]
          tunnel: w453 -> [w468]
          tunnel: w456 -> [w472]
          tunnel: [w470] -> w459
          tunnel: w457 -> [w473]
          tunnel: [w471] -> w460
          n172 = disable-structure shown="FPGA_BUILT==RIO0" {
            disable-tunnel: w473 -> [w480 w487]
            disable-tunnel: w472 -> [w479 w486]
            disable-tunnel: [w478 w485] -> w471
            disable-tunnel: [w477 w484] -> w470
            disable-tunnel: w467 -> [w476 w483]
            disable-tunnel: w468 -> [w475 w482]
            disable-tunnel: [w474 w481] -> w466
            frame condition #0 {
              n173 = xnode "Invoke Method"("FPGA VI Reference In"=w480, "error in"=w479, "Number of Elements"=w476, "Timeout (ms)"=w475) -> ("FPGA VI Reference Out"=w478:T9, "error out"=w477:errorcluster, "Elements Remaining"=w474)  [unwired: 1 out]
            }
            frame condition #1 (active) {
              n174 = xnode "Invoke Method"("FPGA VI Reference In"=w487, "error in"=w486, "Number of Elements"=w483, "Timeout (ms)"=w482) -> ("FPGA VI Reference Out"=w485:T9, "error out"=w484:errorcluster, "Elements Remaining"=w481:u32)  [unwired: 1 out]
            }
          }
          n175 = Wait (ms)(milliseconds to wait=w469) -> ()  [unwired: 1 out]
        }
      }
      frame "FPGA.startId" {
        n176 = Variant To Data(error in=w520, type=enum16{"Axial", "Lateral"}."Axial" ("x"), Variant=w519) -> (data=w518:enum16{"Axial", "Lateral"}, error out=w517:errorcluster)
        n177 = control-ref of="Measured Resp A"() -> (w512:refnum<vi>)
        n178 = control-ref of="Measured Resp Phi"() -> (w513:refnum<vi>)
        n179 = Build Array(w512, w513) -> (w511:refnum<vi>[])
        n180 = for {
          tunnel: w511 -> [w529] mode=indexing
          tunnel: cluster{dbl[], dbl[]} {[], []} ("Value") -> [w528]
          n181 = property on="Property Node" class="XYGraph (strict)"(reference=w529, "Value"=w528) -> ()  [unwired: 1 in, 2 out]
        }
        n182 = case shown="\"Axial\", Default" w518 {
          tunnel: [w535 w541] -> w527
          tunnel: [w534 w538] -> w526
          tunnel: w516 -> [w533 w538]
          tunnel: w517 -> [w532 w540]
          tunnel: w522 -> [w531 w539]
          tunnel: [w531 w536] -> w521
          tunnel: TRUE ("se.sid.start") -> [w530 w537]
          frame "Axial", Default {
            n183 = xnode "Read/Write Control"("FPGA VI Reference In"=w533, "error in"=w532, "sid.p.start"=w530) -> ("FPGA VI Reference Out"=w534:T9, "error out"=w535:errorcluster)
          }
          frame "Lateral" {
            n184 = xnode "Read/Write Control"("FPGA VI Reference In"=w539, "error in"=w540, "se.sid.start"=w537) -> ("FPGA VI Reference Out"=w536:T7, "error out"=w541:errorcluster)
          }
        }
      }
      frame "Buffer" {
        n185 = Variant To Data(error in=w550, type=TRUE, Variant=w549) -> (data=w542:bool, error out=w546:errorcluster)
        n186 = case shown="True" w542 {
          tunnel: [w560 w577] -> w547
          tunnel: w546 -> [w555 w576]
          tunnel: w545 -> [w565 w575]
          tunnel: [w561 w574] -> w544
          frame False {
            # "Remove from the stack"
            n187 = call "FGVHdtServer.vi"("Enum"=EnumFGVHDT."Pop", "error in"=w555) -> ("error out"=w564:errorcluster, "HdtTransferSourceOut"=w554:u8[])  [unwired: 6 in, 2 out]
            n188 = Index Array(array=w554) -> (element=w557:u8)  [unwired: 1 in]
            n189 = xnode ("Read/Write Control")("FPGA VI Reference In"=w565, "error in"=w564) -> ("FPGA VI Reference Out"=w563:T9, "error out"=w562:errorcluster, "hdt.int.p.readParams"=w559:T16)
            n190 = Bundle By Name(cluster=w559, "hdt.int.s.transferSource"=w557) -> (w558:T16)
            n191 = xnode ("Read/Write Control")("FPGA VI Reference In"=w563, "error in"=w562, "hdt.int.p.readParams"=w558) -> ("FPGA VI Reference Out"=w561:T9, "error out"=w560:errorcluster)
          }
          frame True {
            w567 = u8 4 items=["memoryChan1", "memoryChan2", "processVarFixedNoPts", "processVarStream", "systemID"] ("hdt.int.s.transferSource")
            # "Add to the stack"
            n192 = xnode ("Read/Write Control")("FPGA VI Reference In"=w575, "error in"=w576) -> ("FPGA VI Reference Out"=w582:T9, "error out"=w572:errorcluster, "hdt.int.p.readParams"=w581:T16)
            n193 = control-ref of="This VI"() -> (w578:refnum<vi>)
            n194 = property class="VI"(reference=w578, error in=w572) -> (error out=w566:errorcluster, "Name"=w571:string)  [unwired: 1 out]
            n195 = Bundle By Name(cluster=T14 {"OwnerVi"="", "hdt.int.s.transferSource"=2, "Used"=TRUE} ("NewData"), "OwnerVi"=w571, "hdt.int.s.transferSource"=w567, "Used"=TRUE) -> (w568:T14)
            n196 = Bundle By Name(cluster=w581, "hdt.int.s.transferSource"=w567) -> (w580:T16)
            n197 = call "FGVHdtServer.vi"("NewData"=w568, "Enum"=EnumFGVHDT."Push", "error in"=w566) -> ("error out"=w579:errorcluster)  [unwired: 5 in, 3 out]
            n198 = xnode ("Read/Write Control")("FPGA VI Reference In"=w582, "error in"=w579, "hdt.int.p.readParams"=w580) -> ("FPGA VI Reference Out"=w574:T9, "error out"=w577:errorcluster)
          }
        }
      }
      frame "FPGA.readSystemResponse" {
        n199 = local read "System ID Parameters"() -> (w586:T2)
        n200 = local read "PRBS length"() -> (w589:u16)
        n201 = Unbundle By Name(w586) -> ("Repetitions"=w585:u16)
        n202 = for {
          N: w585 -> [w599]
          tunnel: w594 -> [w608]
          tunnel: w589 -> [w607]
          tunnel: [w603] -> w588 mode=concatenating
          tunnel: [w604] -> w593
          tunnel: w592 -> [w602]
          tunnel: [w609] -> w591
          tunnel: w590 -> [w601]
          tunnel: 1000 ("Timeout (ms)") -> [w596]
          i -> [w600]
          stop <- w609 stop-if-true
          n203 = disable-structure shown="FPGA_BUILT==RIO0" {
            disable-tunnel: w608 -> [w616 w623]
            disable-tunnel: w607 -> [w615 w622]
            disable-tunnel: [w614 w621] -> w606
            disable-tunnel: [w613 w620] -> w604
            disable-tunnel: w602 -> [w612 w619]
            disable-tunnel: [w611 w618] -> w609
            disable-tunnel: w596 -> [w610 w617]
            frame condition #0 {
              n204 = xnode "Invoke Method"("FPGA VI Reference In"=w616, "error in"=w612, "Number of Elements"=w615, "Timeout (ms)"=w610) -> ("FPGA VI Reference Out"=w613:T9, "error out"=w611:errorcluster, "Data"=w614:void[])  [unwired: 1 out]
            }
            frame condition #1 (active) {
              n205 = xnode "Invoke Method"("FPGA VI Reference In"=w623, "error in"=w619, "Number of Elements"=w622, "Timeout (ms)"=w617) -> ("FPGA VI Reference Out"=w620:T9, "error out"=w618:errorcluster, "Data"=w621:i16[])  [unwired: 1 out]
            }
          }
          n206 = Increment(x=w600) -> (x+1=w597:i32)
          n207 = Divide(x=w597, y=w599) -> (x/y=→"acquisitionDone":dbl)
          n208 = Build Array(w601, w606) -> (w605:i16[][])
          n209 = Transpose 2D Array(2D array=w605) -> (transposed array=w603:i16[][])
        }
        n210 = Transpose 2D Array(2D array=w588) -> (transposed array=→"Time domain":i16[][])
      }
      frame "USBRio.readSystemResponse" {
        n211 = xnode "Read/Write Control"("FPGA VI Reference In"=w628) -> ("FPGA VI Reference Out"=w624:T9)  [unwired: 1 in, 2 out]
        n212 = local read "System ID Parameters"() -> (w633:T2)
        n213 = local read "PRBS length"() -> (w634:u16)
        n214 = Unbundle By Name(w633) -> ("Repetitions"=w632:u16)
        n215 = for {
          N: w632 -> [w645]
          tunnel: w634 -> [w651]
          tunnel: [w647] -> w625 mode=concatenating
          tunnel: [w648] -> w629
          tunnel: [w638] -> w631
          tunnel: w630 -> [w643]
          tunnel: w624 -> [w642]
          tunnel: w627 -> [w641]
          tunnel: 1000 ("Timeout (ms)") -> [w639]
          i -> [w646]
          stop <- w638 stop-if-true
          n216 = xnode "Invoke Method"("FPGA VI Reference In"=w642, "error in"=w643, "Number of Elements"=w651, "Timeout (ms)"=w639) -> ("FPGA VI Reference Out"=w648:T9, "error out"=w638:errorcluster, "Data"=w650:i16[])  [unwired: 1 out]
          n217 = Increment(x=w646) -> (x+1=w644:i32)
          n218 = Divide(x=w644, y=w645) -> (x/y=w640:dbl)
          n219 = local write "acquisitionDone"(w640) -> ()
          n220 = Build Array(w641, w650) -> (w649:i16[][])
          n221 = Transpose 2D Array(2D array=w649) -> (transposed array=w647:i16[][])
        }
        n222 = Transpose 2D Array(2D array=w625) -> (transposed array=w635:i16[][])
        n223 = local write "Time domain"(w635) -> ()
      }
      frame "FPGA.writeFilter" {
        # "Largest possible coefficient on FPGA"
        # "Hold output to prevent jumps from filter transients"
        # "Give filters a moment to start outputting"
        n224 = Variant To Data(error in=w689, type=cluster{dbl[], dbl[]} {[], []} ("output cluster"), Variant=w690) -> (data=w688:cluster{dbl[], dbl[]}, error out=w694:errorcluster)
        n225 = local write "doControlDesign"(FALSE ("doControlDesign")) -> ()
        n226 = xnode "Read/Write Control"("FPGA VI Reference In"=w679, "error in"=w694, "flt.o.hold"=TRUE) -> ("FPGA VI Reference Out"=w678:T9, "error out"=w677:errorcluster)
        n227 = Unbundle(w688) -> (w668:dbl[], w669:dbl[])
        n228 = Build Array (concatenate)(w668, w669) -> (w667:dbl[])
        n229 = Array Size(array=w669) -> (size(s)=w687:i32)
        n230 = Absolute Value(x=w667) -> (abs(x)=w666:dbl[])
        n231 = Negate(x=w669) -> (-x=w683:dbl[])
        n232 = Divide(x=w687, y=2) -> (x/y=w684:dbl)
        n233 = Greater Or Equal?(x=w666, y=128.0) -> (x >= y?=w664:bool[])
        n234 = for {
          N: 8 -> [_]
          tunnel: w684 -> [w699]
          tunnel: [w698] -> w660 mode=indexing
          i -> [w700]
          n235 = Greater Or Equal?(x=w700, y=w699) -> (x >= y?=w698:bool)
        }
        n236 = Boolean To (0,1)(Boolean=w664) -> (0, 1=w663:i16[])
        n237 = To Unsigned Long Integer(number=w663) -> (unsigned 32bit integer=w653:u32[])
        n238 = Add Array Elements(numeric array=w653) -> (sum=w662:u32)
        n239 = Greater Than 0?(x=w662) -> (x > 0?=w655:bool)
        n240 = Not(x=w655) -> (.not. x?=→"axialFiltersLoaded":bool)
        n241 = Select(t=bool[] [TRUE, TRUE, TRUE, TRUE, TRUE, TRUE, TRUE, TRUE], s=w655, f=w660) -> (s? t:f=w661:bool[])
        n242 = xnode "Read/Write Control"("FPGA VI Reference In"=w678, "error in"=w677, "flt.p.b8x"=w668, "flt.p.anot8x"=w683, "flt.bypass1"=w661) -> ("FPGA VI Reference Out"=w672:T9, "error out"=w670:errorcluster)
        n243 = flat-sequence {
          tunnel: [w696] -> w673
          tunnel: w672 -> [w696]
          tunnel: [w695] -> w671
          tunnel: w670 -> [w695]
          frame #0 {
            n244 = Wait (ms)(milliseconds to wait=u32 10) -> ()  [unwired: 1 out]
          }
        }
        n245 = xnode "Read/Write Control"("FPGA VI Reference In"=w673, "error in"=w671, "flt.o.hold"=FALSE) -> ("FPGA VI Reference Out"=w675:T9, "error out"=w654:errorcluster)
        n246 = Select(t="Warning: Filter coefficients too large! Filters loaded, but not enabled" ("Message"), s=w655, f="Filters written to FPGA" ("Message")) -> (s? t:f=w652:string)
        "Warning" <- w652
        n247 = property on="Warning" class="Str"("Visible"=w655, "Text.Text"=w652) -> ()  [unwired: 2 in, 2 out]
      }
      frame "enableFilters" {
        # "Give filters a moment to start outputting"
        # "Hold output to prevent jumps from filter transient"
        n248 = xnode "Read/Write Control"("FPGA VI Reference In"=w717, "error in"=w718, "flt.o.hold"=TRUE) -> ("FPGA VI Reference Out"=w710:T9, "error out"=w709:errorcluster)
        n249 = local read "Controller Order"() -> (w714:dbl)
        n250 = Divide(x=w714, y=2.0) -> (x/y=w712:dbl)
        n251 = for {
          N: 8 -> [_]
          tunnel: w712 -> [w724]
          tunnel: [w723] -> w708 mode=indexing
          i -> [w725]
          n252 = Greater Or Equal?(x=w725, y=w724) -> (x >= y?=w723:bool)
        }
        n253 = local write "doControlDesign"(FALSE ("doControlDesign")) -> ()
        n254 = xnode "Read/Write Control"("FPGA VI Reference In"=w710, "error in"=w709, "flt.bypass1"=w708) -> ("FPGA VI Reference Out"=w705:T9, "error out"=w707:errorcluster)
        n255 = call "WaitError.vi"("error in (no error)"=w707, "milliseconds to wait"=u32 10) -> ("error out"=w703:errorcluster)  [unwired: 9 in]
        n256 = xnode "Read/Write Control"("FPGA VI Reference In"=w705, "error in"=w703, "flt.o.hold"=FALSE) -> ("FPGA VI Reference Out"=w704:T9, "error out"=w702:errorcluster)
      }
      frame "disableFilters" {
        n257 = local read "Filtering mode"() -> (w726:enum16{"Axial", "Lateral"})
        n258 = case shown="\"Axial\", Default" w726 {
          tunnel: w733 -> [w741 w743]
          tunnel: [w740 w743] -> w732
          tunnel: [w739 w744] -> w731
          tunnel: w728 -> [w738 w745]
          frame "Axial", Default {
            n259 = local write "axialFiltersLoaded"(FALSE ("resetFilters")) -> ()
            n260 = xnode "Read/Write Control"("FPGA VI Reference In"=w741, "error in"=w738, "flt.bypass1"=bool[] [TRUE, TRUE, TRUE, TRUE, TRUE, TRUE, TRUE, TRUE]) -> ("FPGA VI Reference Out"=w740:T9, "error out"=w739:errorcluster)
          }
          frame "Lateral" {
            n261 = local write "lateralFiltersLoaded"(FALSE ("resetFilters")) -> ()
            n262 = call "FGVLateralFilter.vi"("Enum"=Enum."Init", "error in"=w745) -> ("error out"=w744:errorcluster)  [unwired: 5 in, 2 out]
          }
        }
        n263 = local write "resetFilters"(FALSE ("resetFilters")) -> ()
      }
      frame "---- MATLAB -----" {
      }
      frame "MATLAB.identFreqResp" {
        w794 = 0.001  # convertTokHz
        w801 = 0.1  # MinFrequency(kHz)
        # "-30dB minimum"
        n264 = Variant To Data(error in=w760, type=refnum<vi> refnum ("Filtering mode"), Variant=w775) -> (data=w770:refnum<vi>, error out=w769:errorcluster)
        n265 = call <vilib>:"Check if File or Folder Exists.vi"("path"=w791) -> ("file or folder exists?"=w790:bool, "dup path"=w789:path)  [unwired: 8 in, 1 out]
        n266 = property class="Enum (strict)"(reference=w770, error in=w769) -> (error out=w816:errorcluster, "Strings []"=w768:string[], "Value"=w767:enum16{"Axial", "Lateral"})  [unwired: 1 out]
        n267 = case shown="False" w790 {
          tunnel: w789 -> [w821 _]
          frame False {
            n268 = Create Folder(path (use dialog)=w821) -> ()  [unwired: 2 in, 3 out]
          }
          frame True {
          }
        }
        n269 = local read "System ID Parameters"() -> (w800:T2)
        n270 = Index Array(array=w768, index=w767) -> (element=w766:string)
        n271 = local read "Sampling Frequency"() -> (w796:dbl)
        n272 = case shown="True" "Save identification" {
          tunnel: w793 -> [w822 w829]
          tunnel: [w823 w828] -> w763
          tunnel: w816 -> [w823 w824]
          tunnel: w766 -> [_ w825]
          tunnel: [w822 w826] -> w814
          frame False {
          }
          frame True {
            n273 = call "Enqueue Message.vi"("error in"=w824, "Data"=w825, "Message"="saveIdentification", "Queue"=w829) -> ("error out"=w828:errorcluster, "Queue dup."=w826:refnum<queue>)  [unwired: 6 in]
          }
        }
        n274 = Unbundle By Name(w800) -> ("PRBS Order"=w799:u16, "Repetitions"=w798:u16)
        n275 = Reciprocal(x=w796) -> (1/x=w809:dbl)
        n276 = script code="cd(pa)\n\n[i,j]=size(data);\nif( j > i)\n   data = data' ;\nend\nlength_prbs=2^order_prbs-1;\n\nsave data_ident data\n\nudat=data(:,1);\nydat=data(:,2);\nu=udat(1:n_periods*length_prbs);\ny=ydat(1:n_periods*length_prbs);\n\nif mode==0\n  data = detrend(iddata(y,u,Ts));\n  w=0:2*pi/(Ts*length_prbs):(length_prbs-1)*2*pi/(Ts*length_prbs);\n  G_freqresp = spa(data,700,w(1:(length_prbs-1)/2));\nelseif mode==1\n  w=0:2*pi/(Ts*length_prbs):(length_prbs-1)*2*pi/(Ts*length_prbs);\n  U1=fft(u);\n  Y1=fft(y);\n  g=Y1(1:n_periods:end)./U1(1:n_periods:end);\n  G_freqresp=frd(g(1:(length_prbs-1)/2),w(1:(length_prbs-1)/2));\nend\n\nsave G_freqresp G_freqresp\n\n[mag,phase,w] = bode(G_freqresp);\nf = (w/(2*pi))';\nmag = mag2db(mag(:)');\n\nphase = phase(:)';\n\nstatus = 'Done!';"("??"=w763, "Ts"=w809, "n_periods"=w798, "order_prbs"=w799, "pa"=w791, "data"=w810, "mode"=w767) -> ("??"=w815:errorcluster, "mag"=w788:dbl[], "phase"=w802:dbl[], "f"=w803:dbl[])  [unwired: 1 out]
        n277 = Bundle(w803, w788) -> (→"Measured Resp A":cluster{dbl[], dbl[]})  [unwired: 1 in]
        n278 = Bundle(w803, w802) -> (→"Measured Resp Phi":cluster{dbl[], dbl[]})  [unwired: 1 in]
        n279 = Array Size(array=w803) -> (size(s)=w806:i32)
        n280 = Decrement(x=w806) -> (x-1=w805:i32)
        n281 = Delete From Array(array=w788, length=20, index=0) -> (array with subset deleted=w779:dbl[])  [unwired: 1 out]
        n282 = Index Array(array=w803, index=w805) -> (element=w804:dbl)
        n283 = Array Max & Min(array=w779) -> (max value=w787:dbl, min value=w784:dbl)  [unwired: 2 out]
        n284 = Multiply(x=w804, y=w794) -> (x*y=w795:dbl)
        n285 = control-ref of="Measured Resp A"() -> (w774:refnum<vi>)
        n286 = control-ref of="Nominal Response A"() -> (w773:refnum<vi>)
        n287 = Bundle By Name(cluster=T11 {"Message"="Feedback.PIDUpdate", "Données de message"=variant} ("Cluster Message"), "Données de message"=FALSE) -> (w758:T11)
        n288 = Add(x=2.0, y=w787) -> (x+y=w785:dbl)
        n289 = property on="Measured Resp A" class="XYGraph (strict)"("XScale.Minimum"=w801, "XScale.Maximum"=w795) -> ()  [unwired: 2 in, 2 out]
        n290 = property on="Measured Resp Phi" class="XYGraph (strict)"("XScale.Minimum"=w801, "XScale.Maximum"=w795, "YScale.Maximum"=180.0 ("Y Scale.Range:Maximum"), "YScale.Minimum"=-360.0 ("Y Scale.Range:Minimum")) -> ()  [unwired: 2 in, 2 out]
        n291 = In Range and Coerce(upper limit=0.0, x=w784, lower limit=-30.0) -> (coerced(x)=w782:dbl)  [unwired: 1 out]
        n292 = Round Toward +Infinity(x=w785) -> (ceil(x): smallest int >= x=w778:dbl)
        n293 = Obtain Queue(name (unnamed)="ZController", element data type=T11 {"Message"="", "Données de message"=variant} ("Cluster Message"), error in (no error)=w815) -> (queue out=w817:refnum<queue>, error out=w755:errorcluster)  [unwired: 2 in, 1 out]
        n294 = Round Toward -Infinity(1:w782) -> (0:w776:dbl)
        n295 = Build Array(w774, w773) -> (w772:refnum<vi>[])
        n296 = for {
          tunnel: w778 -> [w820]
          tunnel: w776 -> [w819]
          tunnel: w772 -> [w818] mode=indexing
          n297 = property on="Property Node" class="XYGraph"(reference=w818, "YScale.Maximum"=w820, "YScale.Minimum"=w819) -> ()  [unwired: 1 in, 2 out]
        }
        n298 = Enqueue Element(queue=w817, element=w758, error in (no error)=w755) -> (error out=w753:errorcluster)  [unwired: 1 in, 2 out]
        n299 = call "Enqueue Message.vi"("error in"=w753, "Message"="MATLAB.cleanUp", "Queue"=w814) -> ("error out"=w761:errorcluster)  [unwired: 7 in, 1 out]
      }
      frame "MATLAB.cleanUp" {
        n300 = script code="clear all"("??"=w831) -> ("??"=w830:errorcluster)
      }
      frame "saveIdentification" {
        # "Save images of frequency response"
        n301 = local read "axialFiltersLoaded"() -> (w843:bool)
        n302 = local read "idSourceName"() -> (w840:string)
        n303 = Variant To Data(error in=w879, type="" ("element"), Variant=w878) -> (data=w839:string, error out=w886:errorcluster)
        n304 = local read "System ID Parameters"() -> (w866:T2)
        n305 = local read "Sampling Frequency"() -> (w864:dbl)
        n306 = local read "PRBS length"() -> (w865:u16)
        n307 = xnode "Read/Write Control"("FPGA VI Reference In"=w852) -> ("flt.p.b8x"=w851:fxp<+/-,24,8>[], "flt.p.anot8x"=w850:fxp<+/-,24,8>[], "flt.bypass1"=w849:bool[])  [unwired: 1 in, 2 out]
        n308 = Select(t="filtered" ("string"), s=w843, f="unFiltered" ("string")) -> (s? t:f=w845:string)
        n309 = Build Path(base path=w860, name or relative path="idParams.xml" ("text")) -> (appended path=w854:path)
        n310 = Format Date/Time String(time format string (%c)="%Y-%m-%d_%H%M%S_") -> (date/time string=w877:string)  [unwired: 2 in]
        n311 = case shown="True" w843 {
          tunnel: string[] ["G_freqresp.mat", "data_ident.mat"] -> [w888 w891]
          tunnel: [w888 w890] -> w846
          frame False {
          }
          frame True {
            n312 = Build Array (concatenate)(w891, string[] ["K_designed.mat"] ("array")) -> (w890:string[])
          }
        }
        n313 = Concatenate Strings(w877, w839, "Id_" ("string"), w840, w845, ".zip" ("string")) -> (w874:string)
        n314 = control-ref of="Measured Resp Phi"() -> (w848:refnum<vi>)
        n315 = control-ref of="Measured Resp A"() -> (w847:refnum<vi>)
        n316 = Bundle("System ID Parameters"=w866, "PRBS length"=w865, "Sampling Frequency"=w864, "flt.p.b8x"=w851, "flt.p.anot8x"=w850, "flt.bypass1"=w849) -> (w863:T17)  [unwired: 1 in]
        n317 = call "FGVSavingParameters.vi"("Enum"=Enum."Read") -> ("pathOut"=w875:path)  [unwired: 7 in, 3 out]
        n318 = Flatten To XML(anything=w863) -> (xml string=w861:string)
        n319 = Build Path(base path=w875, name or relative path=w874) -> (appended path=w873:path)
        n320 = Build Array(w847, w848) -> (w867:refnum<vi>[])
        n321 = Write to Text File(file (use dialog)=w854, text=w861, error in=w886) -> (error out=w855:errorcluster)  [unwired: 1 in, 2 out]
        n322 = for {
          tunnel: w867 -> [w908] mode=indexing
          tunnel: w860 -> [w904]
          tunnel: [w901] -> w856 mode=indexing
          tunnel: w855 -> [w909]
          tunnel: [w906] -> w887
          tunnel: ".png" ("string") -> [w896]
          tunnel: refnum<vi> refnum ("Measured Resp A") -> [w895]
          n323 = invoke on="Invoke Node" class="XYGraph (strict)" method="Get Image"(reference=w908, error in=w909) -> (reference out=w900:refnum<vi>, error out=w898:errorcluster, "image data"=w907:T18)  [unwired: 4 in, 3 out]
          n324 = To More Specific Class(target class=w895, reference=w900, error in=w898) -> (specific class reference=w899:refnum<vi>, error out=w897:errorcluster)
          n325 = property class="XYGraph (strict)"(reference=w899, error in=w897) -> (error out=w906:errorcluster, "Label.Text"=w905:string)  [unwired: 1 out]
          n326 = Concatenate Strings(w905, w896) -> (w903:string)
          n327 = Build Path(base path=w904, name or relative path=w903) -> (appended path=w902:path)
          n328 = call <vilib>:"Write PNG File.vi"("image data"=w907, "path to PNG file"=w902) -> ("path"=w901:path)  [unwired: 8 in, 1 out]
        }
        n329 = for {
          tunnel: w860 -> [w894]
          tunnel: w846 -> [w893] mode=indexing
          tunnel: [w892] -> w857 mode=indexing
          n330 = Build Path(base path=w894, name or relative path=w893) -> (appended path=w892:path)
        }
        n331 = Build Array (concatenate)(w857, w856, w854) -> (w858:path[])
        n332 = call <vilib>:"New Zip File.vi"("error in (no error)"=w887, "target"=w873) -> ("error out"=w871:errorcluster, "zip file out"=w872:i64)  [unwired: 3 in, 1 out]
        n333 = for {
          shift-right: [w915] -> w870
          shift-left: w872 -> [w917]
          tunnel: w858 -> [w913] mode=indexing
          tunnel: w871 -> [w916]
          tunnel: [w914] -> w869
          n334 = Strip Path(path=w913) -> (name=w912:string)  [unwired: 1 out]
          n335 = Build Path(base path=path "", name or relative path=w912) -> (appended path=w910:path)
          n336 = call <vilib>:"Add File to Zip.vi"("error in (no error)"=w916, "destination path in zip"=w910, "source file path"=w913, "zip file in"=w917) -> ("error out"=w914:errorcluster, "zip file out"=w915:i64)  [unwired: 6 in]
        }
        n337 = call <vilib>:"Close Zip File.vi"("error in (no error)"=w869, "zip file in"=w870) -> ("error out"=w868:errorcluster)  [unwired: 5 in]
      }
      frame "ControlDesign.clearPlots" {
        n338 = control-ref of="Nominal Response A"() -> (w920:refnum<vi>)
        n339 = control-ref of="Nominal Response Phi"() -> (w919:refnum<vi>)
        n340 = Build Array(w920, w919) -> (w921:refnum<vi>[])
        n341 = for {
          tunnel: w921 -> [w929] mode=indexing
          tunnel: cluster{dbl[], dbl[]}[] [] ("Value") -> [w928]
          n342 = property on="Property Node" class="XYGraph (strict)"(reference=w929, "Value"=w928) -> ()  [unwired: 1 in, 2 out]
        }
      }
      frame "ControlDesign" {
        w945 = 0.5
        n343 = local read "Sampling Frequency"() -> (w940:dbl)
        n344 = Reciprocal(x=w940) -> (1/x=w944:dbl)
        n345 = script code="%go to current folder\ncd(pa)\naddpath ../LAC\n\nload G_freqresp\n\norder_x = order_y;\n%[K,Ld,status] =controldesign_z_fun_I_dataCompress_poleHack(G_freqresp, Ts, fc, order_x, order_y,0);\n[K,Ld,status] = controldesign_z_fun_I(G_freqresp, Ts, fc, order_x, order_y,0);\nsave K_designed K Ts\n\nif strcmp(status,'Converged!')\n   [Kp, Ki, K_filt_sos_num, K_filt_sos_den] = separate_I_filter_z(K)  \n   K_filt_sos_num = K_filt_sos_num';\n   K_filt_sos_den = K_filt_sos_den';\nelse \n   [Knum_arr, Kden_arr] = [0 0];\n   Kp=0;\n   Ki=0;\nend\n\nG_freqresp.Ts=Ts\n\nz = tf('z',Ts);\n[T_mag, T_phase, T_w] = bode( feedback(G_freqresp*K/(z-1), 1) );\n[Ld_mag, Ld_phase, Ld_w] = bode( feedback(Ld, 1), T_w );\n\nLd_f = (Ld_w/(2*pi))';\nLd_mag = mag2db(Ld_mag(:)');\n\nLd_phase = Ld_phase(:)';\n\nT_f = (T_w/(2*pi))';\nT_mag = mag2db(T_mag(:)');\n\nT_phase = T_phase(:)';"("??"=w935, "pa"=w937, "fc"="Desired bandwidth", "Ts"=w944, "order_y"="Controller Order") -> ("??"=w934:errorcluster, "K_filt_sos_num"=w963:dbl[], "K_filt_sos_den"=w962:dbl[], "Kp"=→"Kp":dbl, "Ki"=→"Ki":dbl, "T_mag"=w951:dbl[], "T_phase"=w949:dbl[], "T_f"=w950:dbl[], "Ld_f"=w948:dbl[], "Ld_mag"=w947:dbl[], "Ld_phase"=w946:dbl[])  [unwired: 1 out]
        n346 = Bundle(w963, w962) -> (w961:cluster{dbl[], dbl[]})  [unwired: 1 in]
        n347 = Bundle(w950, w951) -> (w960:cluster{dbl[], dbl[]})  [unwired: 1 in]
        n348 = Bundle(w950, w949) -> (w958:cluster{dbl[], dbl[]})  [unwired: 1 in]
        n349 = Bundle(w948, w947) -> (w959:cluster{dbl[], dbl[]})  [unwired: 1 in]
        n350 = Bundle(w948, w946) -> (w957:cluster{dbl[], dbl[]})  [unwired: 1 in]
        n351 = call "Enqueue Message.vi"("error in"=w934, "Data"=w961, "Message"="FPGA.writeFilter", "Queue"=w970) -> ("error out"=w932:errorcluster, "Queue dup."=w933:refnum<queue>)  [unwired: 6 in]
        n352 = Build Array(w960, w959) -> (→"Nominal Response A":cluster{dbl[], dbl[]}[])
        n353 = Build Array(w958, w957) -> (→"Nominal Response Phi":cluster{dbl[], dbl[]}[])
        n354 = Array Size(array=w950) -> (size(s)=w954:i32)
        n355 = Decrement(x=w954) -> (x-1=w955:i32)
        n356 = call "Enqueue Message.vi"("error in"=w932, "Message"="MATLAB.cleanUp", "Queue"=w933) -> ("error out"=w931:errorcluster)  [unwired: 7 in, 1 out]
        n357 = Index Array(array=w950, index=w955) -> (element=w956:dbl)
        n358 = Multiply(x=w956, y=0.001) -> (x*y=w939:dbl)
        n359 = property on="Nominal Response A" class="XYGraph (strict)"("XScale.Minimum"=w945, "XScale.Maximum"=w939) -> ()  [unwired: 2 in, 2 out]
        n360 = property on="Nominal Response Phi" class="XYGraph (strict)"("XScale.Minimum"=w945, "XScale.Maximum"=w939) -> ()  [unwired: 2 in, 2 out]
      }
      frame "MakeLateralFilter" {
        n361 = local read "Sampling Frequency"() -> (w988:dbl)
        n362 = local read "Desired bandwidth"() -> (w987:dbl)
        n363 = Reciprocal(x=w988) -> (1/x=w991:dbl)
        n364 = script code="%go to current folder\ncd(pa)\naddpath ../LAC\n\nload G_freqresp\n\n[K,Ld,status] = controldesign_x_prbs(G_freqresp, Ts, fc);\n\n[Ksos,Kk] = tf2sos(K.num{1},K.den{1})\nKsos_num = Ksos(:,1:3);\nKsos_den = Ksos(:,4:6);\n\nclear Kz\nclear Kp\nfor i=1:size(Ksos_num,1)\n Kz(i,:) = roots(Ksos_num(i,:));\n Kp(i,:) = roots(Ksos_den(i,:));\nend\n\nK_lateralfilter = K;\nsave K_lateralfilter K_lateralfilter;\n\nG_freqresp.Ts=Ts\n[L_mag, L_phase, L_w] = bode(K*G_freqresp)\n\nL_f = (L_w/(2*pi))';\nL_mag = mag2db(L_mag(:)');\n\nL_phase = L_phase(:)';"("pa"=w972, "fc"=w987, "Ts"=w991) -> ("Kz"=w982:cdb[][], "Kp"=w981:cdb[][], "Kk"=w971:dbl, "L_f"=w974:dbl[], "L_mag"=w979:dbl[], "L_phase"=w973:dbl[])  [unwired: 1 in, 1 out]
        n365 = local read "Sampling Frequency"() -> (w984:dbl)
        n366 = Bundle(w974, w979) -> (w978:cluster{dbl[], dbl[]})  [unwired: 1 in]
        n367 = Bundle(w974, w973) -> (w976:cluster{dbl[], dbl[]})  [unwired: 1 in]
        n368 = flat-sequence {
          tunnel: w971 -> [_]
          frame #0 {
            n369 = local write "doControlDesign"(FALSE ("doLatFilterDesign")) -> ()
            "lateralFiltersLoaded" <- TRUE ("lateralFiltersLoaded")
          }
        }
        n370 = Build Array(w978) -> (w977:cluster{dbl[], dbl[]}[])
        n371 = Build Array(w976) -> (w975:cluster{dbl[], dbl[]}[])
        n372 = local write "Nominal Response A"(w977) -> ()
        n373 = local write "Nominal Response Phi"(w975) -> ()
        n374 = Reciprocal(x=w984) -> (1/x=w983:dbl)
        n375 = Bundle(w983, w982, w981, w971) -> (w980:cluster{dbl, cdb[][], cdb[][], dbl})  [unwired: 1 in]
        n376 = call "FGVLateralFilter.vi"("Enum"=Enum."Write", "ZPK input cluster"=w980, "Filter valid input"=TRUE) -> ()  [unwired: 4 in, 3 out]
      }
      frame "Exit" {
        n377 = Release Queue(queue=w1006, error in (no error)=w1004) -> (error out=w1003:errorcluster)  [unwired: 1 in, 2 out]
      }
      frame Default {
        n378 = Format Into String(format string="The message\"%s\" received in the gestion loop is not valid" ("Texte de message d'erreur inconnu"), w1015) -> (resulting string=w1012:string)  [unwired: 2 in, 1 out]
        n379 = call <vilib>:"Error Cluster From Error Code.vi"("error message (\"\")"=w1012, "error code (0)"=1 ("code d'erreur (0)")) -> ("error out"=w1013:errorcluster)  [unwired: 7 in]
      }
    }
    n380 = Unbundle By Name(w85) -> ("status"=w83:bool)
    n381 = Select(t="NOT finished", s=w83, f=" finished") -> (s? t:f=w81:string)
    n382 = Concatenate Strings(w87, w81) -> (w86:string)
    n383 = property on="Message" class="Str"(error in=w85, "Value"=w86) -> ()  [unwired: 1 in, 2 out]
  }
  n384 = Merge Errors(w9, w10) -> (w11:errorcluster)
  n385 = call <vilib>:"Simple Error Handler.vi"("error in (no error)"=w11) -> ()  [unwired: 4 in, 5 out]
